vi "generateTriWave_fromAOparameters.vi"(0 "AO params":T1) -> (1 "Waveform":waveform(dbl), 2 "wfsize":i32)   [LabVIEW 2015]
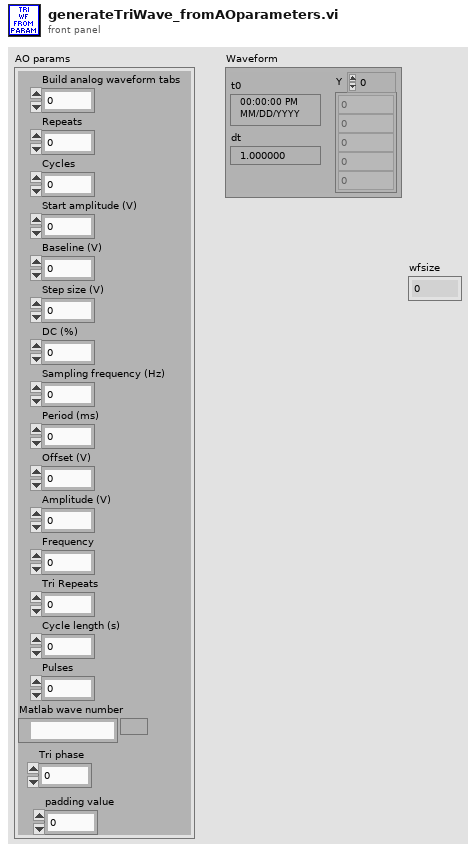
[diagram p1: front panel]
types:
  T1 = cluster{"Build analog waveform tabs":dbl, "Repeats":dbl, "Cycles":dbl, "Start amplitude (V)":dbl, "Baseline (V)":dbl, "Step size (V)":dbl, "DC (%)":dbl, "Sampling frequency (Hz)":dbl, "Period (ms)":dbl, "Offset (V)":dbl, "Amplitude (V)":dbl, "Frequency":dbl, "Tri Repeats":dbl, "Cycle length (s)":dbl, "Pulses":dbl, "Matlab wave number":path, "Tri phase":dbl, "padding value":dbl}
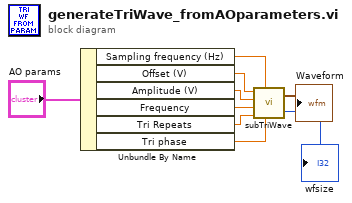
[diagram p0: block diagram]
diagram:
  n1 = Unbundle By Name("AO params") -> ("Sampling frequency (Hz)"=w7:dbl, "Offset (V)"=w6:dbl, "Amplitude (V)"=w5:dbl, "Frequency"=w4:dbl, "Tri Repeats"=w3:dbl, "Tri phase"=w2:dbl)
  n2 = call "subTriWave.vi"("Tri Phase (s)"=w2, "Sampling frequency (Hz)"=w7, "Tri Repeats"=w3, "Frequency"=w4, "Amplitude (V)"=w5, "Offset (V)"=w6) -> ("wfsize"=→"wfsize":i32, "signal out"=→"Waveform":waveform(dbl))
